vi "mmW RecieveCommand.vi"(0 "reference in":refnum<class "ZMQ_mmWave.lvclass">, 11 "error in (no error)":errorcluster) -> (3 "Valid message?":bool, 4 "reference out":refnum<class "ZMQ_mmWave.lvclass">, 6 "command out":T1, 8 "multipart message":string[](array[string]), 14 "timed out?":bool, 15 "error out":errorcluster)   [LabVIEW 2019, in "CommandResponse communication.lvlib" / "ZMQ_mmWave.lvclass"]
doc: "Recieve mmW command:\n- command enum\n- parameters json\n- data (variant)"
uses:
  ZMQ_mmWave.lvclass
  C:/Barkhausen mmWave radar/Development/LV/Barkhausen mmWave hardware control/Host/Intertarget communication/ZMQ_slave_class/ZMQ_slave.lvclass
  mmw_command_lib/src_LabVIEW/mmW_commands/TypeDefs/commands.ctl
  Host/Intertarget communication/ZMQ_slave_class/ZMQ_slave.lvclass
  <vilib>/addons/zeromq/zmq_socket.lvclass
  mmw_command_lib/src_LabVIEW/mmW_commands/mmW_commands.lvlib
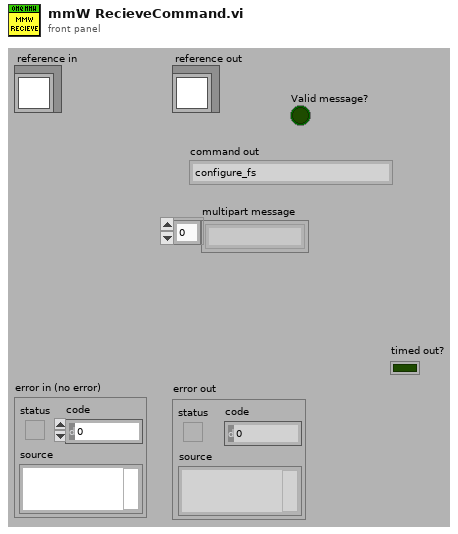
[diagram p1: front panel]
types:
  T1 = typedef "mmW_commands.lvlib/commands.ctl" = enum16{"configure_fs", "configure_rf", "configure_trigger", "equalization_enable", "equalization_start", "lo_sync_enable", "equalization_stop", "get_instrument_status", "get_versions", "initialize_hw", "pop_rx", "set_log_level", "Shutdown", "start", "start_instrument_app", "stop", "trans", "transceive", "trigger_burst", "trigger_sync_enable", "Write TX", "resp_generic", "resp_waveform", "send_trigger", "fetch", "transceive2"}
  T2 = typedef "CommandResponse communication.lvlib/ZMQ_slave.lvclass/ObjectAttributes.ctl" = cluster{"ZMQ context":refnum<class "zmq_context.lvclass">, "ZMQ socket":refnum<class "zmq_socket.lvclass">, "endpoint":string}
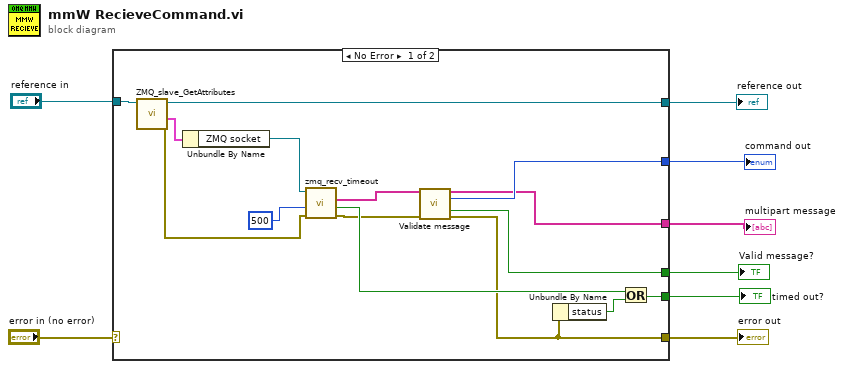
[diagram p0: block diagram]
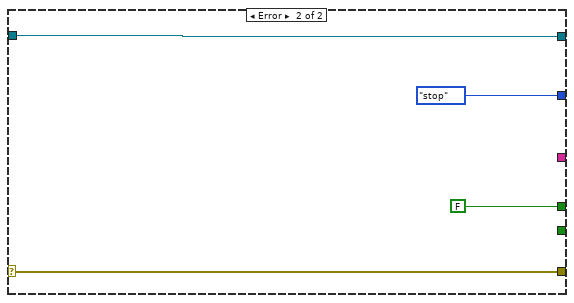
[diagram p2: hidden frame]
diagram:
  n1 = case shown="No Error" "error in (no error)" {
    selector: "error in (no error)" -> [_ w27]
    tunnel: [w11 w27] -> w7
    tunnel: [w23 w26] -> w5
    tunnel: "reference in" -> [w21 w26]
    tunnel: [w10 _] -> w4
    tunnel: [w14 commands."stop" ("command out")] -> w3
    tunnel: [w13 FALSE ("Valid message?")] -> w2
    tunnel: [w12 _] -> w1
    frame No Error {
      n2 = call "ZMQ_slave_GetAttributes.vi"("reference in"=w21) -> ("error out"=w18:errorcluster, "attributes"=w22:T2, "reference out"=w23:refnum<class "ZMQ_mmWave.lvclass">)  [unwired: 7 in, 1 out]
      n3 = Unbundle By Name(w22) -> ("ZMQ socket"=w19:refnum<class "zmq_socket.lvclass">)
      n4 = call <vilib>:"zmq_recv_timeout.vi"("error in"=w18, "timeout (ms)"=u32 500, "socket in"=w19) -> ("error out"=w15:errorcluster, "timeout?"=w17:bool, "parts"=w16:string[])  [unwired: 1 in, 1 out]
      n5 = call "Validate message.vi"("multipart message in"=w16, "error in (no error)"=w15) -> ("multipart message out"=w12:string[], "command out"=w14:T1, "Valid message?"=w13:bool, "error out"=w11:errorcluster)  [unwired: 8 in, 2 out]
      n6 = Unbundle By Name(w11) -> ("status"=w9:bool)
      n7 = Or(x=w17, y=w9) -> (x .or. y?=w10:bool)
    }
    frame Error {
    }
  }
  "error out" <- w7
  "reference out" <- w5
  "timed out?" <- w4
  "Valid message?" <- w2
  "command out" <- w3
  "multipart message" <- w1
